vi "writeImagenDataInImagenTable.vi"(8 "error in":errorcluster, 11 "dataToWrite":T1) -> (0 "error out":errorcluster)   [LabVIEW 2014]
uses:
  <vilib>/addons/database/Connection.llb/DB Tools Open Connec (String).vi
  <vilib>/addons/database/NI_Database_API.lvlib
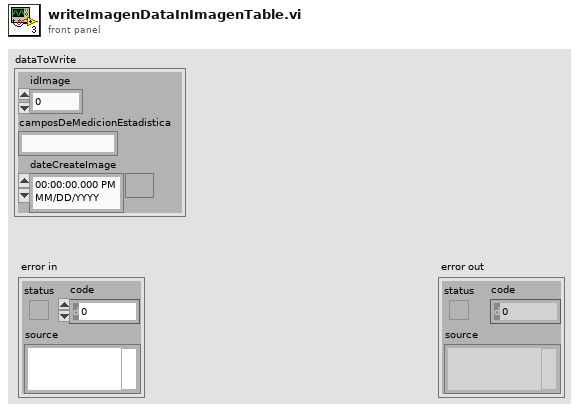
[diagram p1: front panel]
types:
  T1 = cluster{"idImage":dbl, "camposDeMedicionEstadistica":string, "dateCreateImage":timestamp}
  T2 = typedef "NI_Database_API.lvlib/Conn ObjectReference.ctl" = refnum<k1>
  T3 = typedef "NI_Database_API.lvlib/DB Tools DataTypes.ctl" = enum16{"String", "Long (I32)", "Single (SGL)", "Double (DBL)", "Date/Time", "Binary"}
  T4 = cluster{"name":string, "database data type":T3, "defined size":i32}[]
  T5 = cluster{string, "camposDeMedicion":string, "date/time string":string}
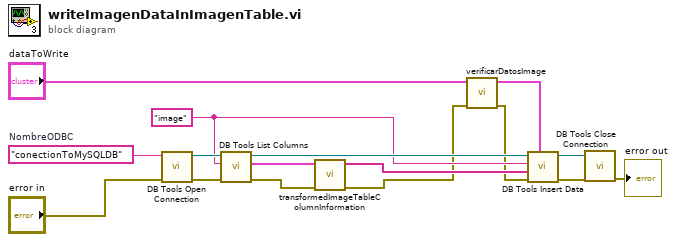
[diagram p0: block diagram]
diagram:
  w11 = "image"
  w16 = "conectionToMySQLDB"  # NombreODBC
  n1 = call-poly <vilib>:"DB Tools Open Connection.vi"("error in (no error)"="error in", "connection information"=w16) -> ("error out"=w14:errorcluster, "connection reference"=w15:T2)  [unwired: 6 in]
  n2 = call <vilib>:"DB Tools List Columns.vi"("error in (no error)"=w14, "table"=w11, "connection reference"=w15) -> ("error out"=w2:errorcluster, "column information"=w6:T4, "connection reference out"=w12:T2)  [unwired: 1 in, 1 out]
  n3 = call "transformedImageTableColumnInformation.vi"("error in"=w2, "columnInformationReading"=w6) -> ("error out"=w4:errorcluster, "columnInformationReadingTransformed"=w5:string[])  [unwired: 8 in]
  n4 = call "verificarDatosImage.vi"("error in"=w4, "dataToWrite"="dataToWrite") -> ("error out"=w1:errorcluster, "dataToWriteModify"=w10:T5)  [unwired: 8 in]
  n5 = call <vilib>:"DB Tools Insert Data.vi"("data"=w10, "error in (no error)"=w1, "columns"=w5, "table"=w11, "connection reference"=w12) -> ("error out"=w9:errorcluster, "connection reference out"=w8:T2)  [unwired: 5 in]
  n6 = call <vilib>:"DB Tools Close Connection.vi"("error in (no error)"=w9, "connection reference"=w8) -> ("error out"=→"error out":errorcluster)  [unwired: 5 in]
